vi "TCPGetVariableSets.vi"(1 "error in (no error)":errorcluster, 4 "connection ID":refnum<k5>) -> ()   [LabVIEW 2013]
uses:
  FBVarSet.ctl
  FBVar.ctl
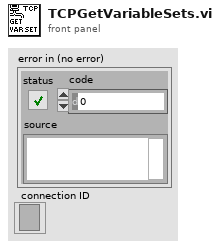
[diagram p1: front panel]
types:
  T1 = typedef "FBVarSet.ctl" = T2[]
  T2 = typedef "FBVar.ctl" = cluster{"Name":string, "Change DV":bool, "Default Value":dbl, "Change SF":bool, "Sequence Function":string, "Change II":bool, "Inform Igor":bool, "Change Seq.":bool, "Sequence":bool, "Change SV":bool, "String Value":string}
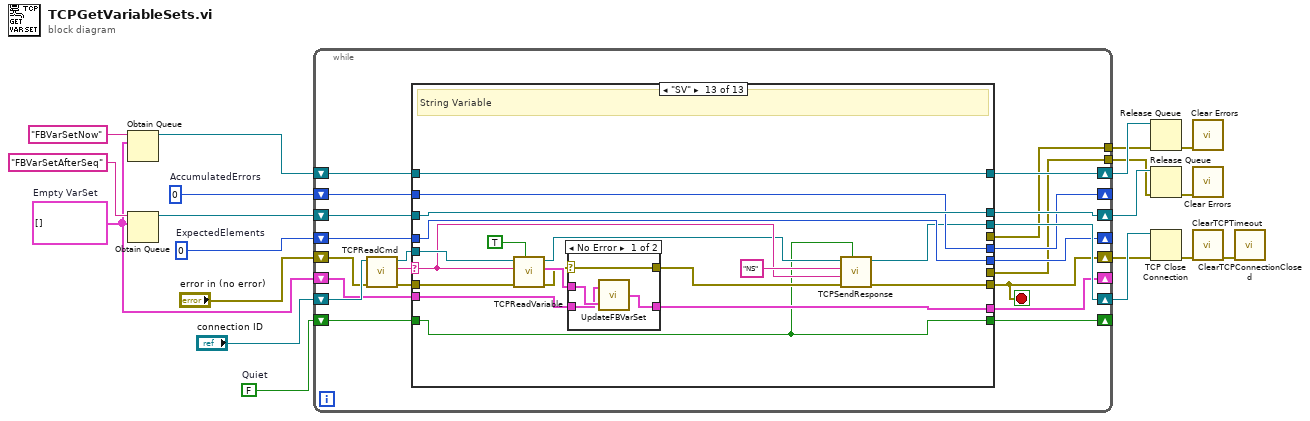
[diagram p0: block diagram]
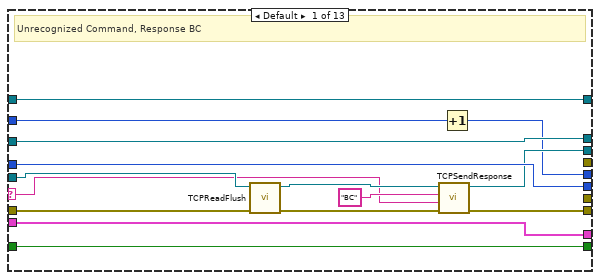
[diagram p2: hidden frame]
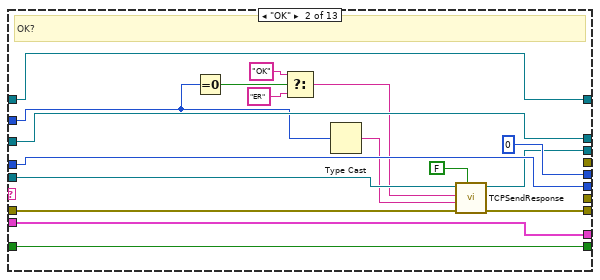
[diagram p3: hidden frame]
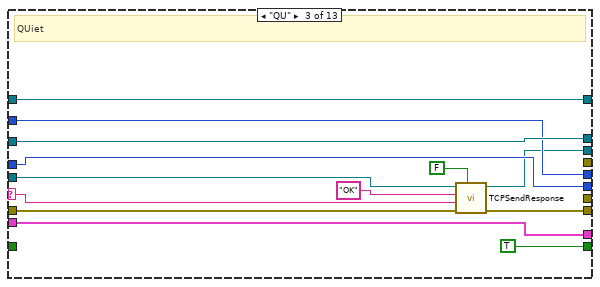
[diagram p4: hidden frame]
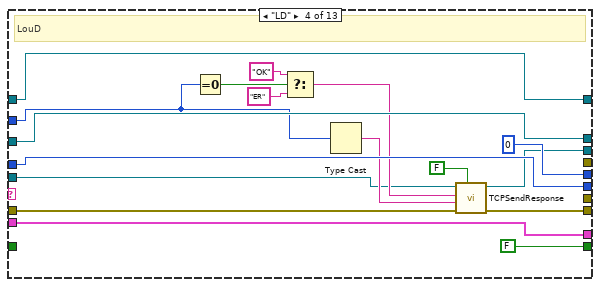
[diagram p5: hidden frame]
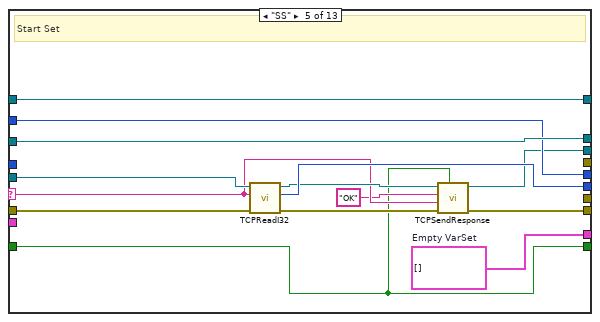
[diagram p6: hidden frame]
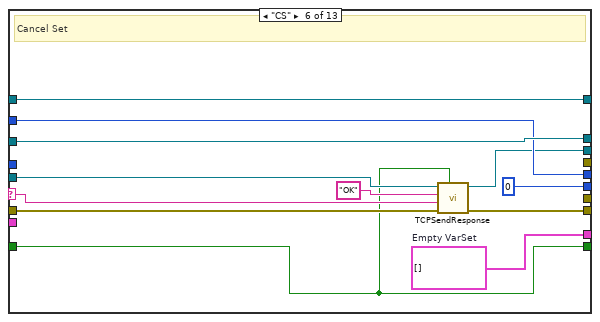
[diagram p7: hidden frame]
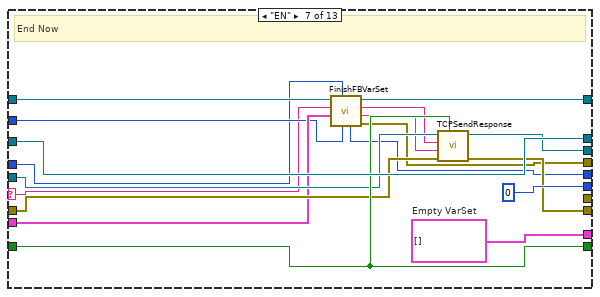
[diagram p8: hidden frame]
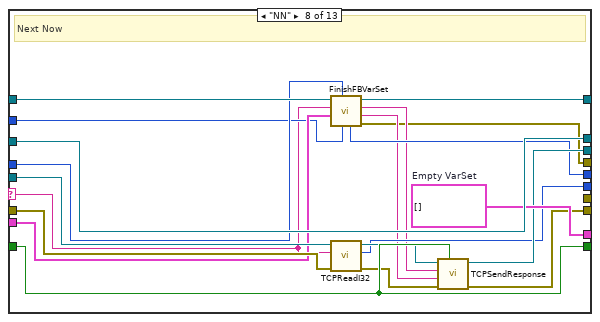
[diagram p9: hidden frame]
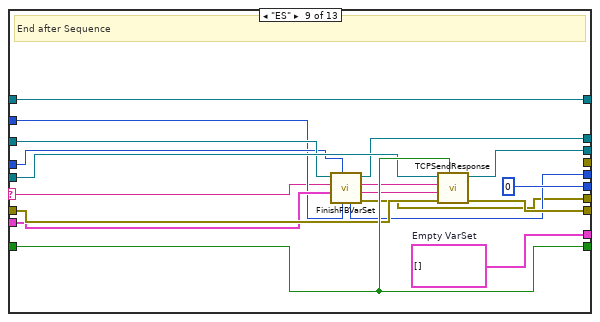
[diagram p10: hidden frame]
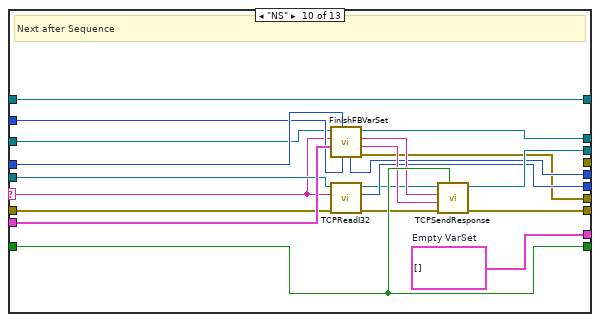
[diagram p11: hidden frame]
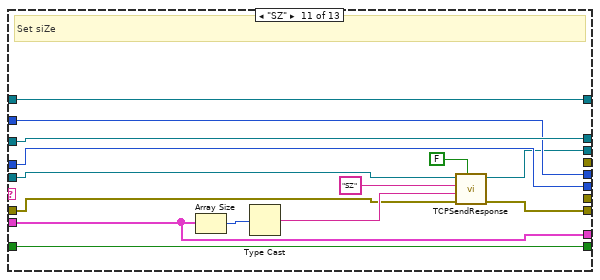
[diagram p12: hidden frame]
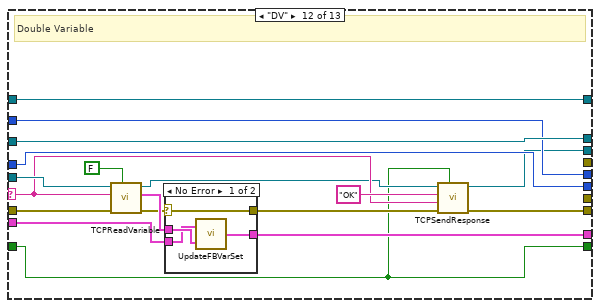
[diagram p13: hidden frame]
diagram:
  w3 = FALSE  # Quiet
  w4 = 0  # AccumulatedErrors
  w6 = T1 []  # Empty VarSet
  w5 = 0  # ExpectedElements
  n1 = Obtain Queue(name (unnamed)="FBVarSetNow", element data type=w6) -> (queue out=w17:refnum<queue>)  [unwired: 3 in, 2 out]
  n2 = Obtain Queue(name (unnamed)="FBVarSetAfterSeq", element data type=w6) -> (queue out=w11:refnum<queue>)  [unwired: 3 in, 2 out]
  n3 = while {
    shift-right: [w35] -> w20
    shift-left: "connection ID" -> [w41]
    shift-right: [w36] -> w16
    shift-left: w17 -> [w39]
    shift-right: [w23] -> w8
    shift-left: "error in (no error)" -> [w32]
    shift-right: [w28] -> _
    shift-left: w5 -> [w29]
    shift-right: [w38] -> w9
    shift-left: w11 -> [w40]
    shift-right: [w30] -> _
    shift-left: w6 -> [w31]
    shift-right: [w26] -> _
    shift-left: w4 -> [w27]
    shift-right: [w24] -> _
    shift-left: w3 -> [w25]
    tunnel: [w22] -> w2
    tunnel: [w21] -> w1
    stop <- w23 stop-if-true
    n4 = call "TCPReadCmd.vi"("error in (no error)"=w32, "connection ID"=w41) -> ("error out"=w33:errorcluster, "Command Code"=w37:string, "connection ID out"=w34:refnum<k5>)  [unwired: 7 in]
    n5 = case shown="\"SV\"" w37 {
      selector: w37 -> [w44 _ w74 _ w106 w125 w131 w149 w171 w188 _ w223 w247]
      tunnel: w40 -> [w56 w73 w86 w103 w117 w129 w147 w167 w176 w195 w219 w237 w261]
      tunnel: w39 -> [w55 w72 w85 w102 w116 w128 w138 w156 w178 w196 w218 w236 w260]
      tunnel: [w56 w73 w86 w103 w117 w129 w147 w167 w175 w194 w219 w237 w261] -> w38
      tunnel: [w55 w72 w85 w102 w116 w128 w137 w155 w178 w196 w218 w236 w260] -> w36
      tunnel: [w47 w61 w78 w88 w108 w121 w143 w164 w182 w200 w208 w221 w245] -> w35
      tunnel: w34 -> [w53 w62 w79 w92 w112 w123 w141 w159 w180 w190 w209 w228 w252]
      tunnel: w33 -> [w54 w63 w80 w91 w113 w126 w140 w158 w179 w193 w212 w227 w251]
      tunnel: [w48 w60 w77 w87 w107 w120 w144 w165 w183 w201 w211 w224 w249] -> w23
      tunnel: w31 -> [w52 w71 w84 w101 _ _ w139 w157 w177 w204 w206 w232 w256]
      tunnel: [w52 w71 w84 w101 w114 w119 w146 w166 w185 w205 w206 w231 w255] -> w30
      tunnel: w29 -> [w51 w70 w83 w100 _ _ w132 w154 w174 w203 w217 w235 w259]
      tunnel: [w51 w70 w83 w100 w111 0 ("I32 value") 0 ("I32 value") w160 0 ("I32 value") w191 w217 w235 w259] -> w28
      tunnel: w27 -> [w43 w67 w82 w90 w115 w127 w133 w153 w172 w202 w216 w234 w258]
      tunnel: [w42 0 ("AccumulatedErros") w82 0 ("AccumulatedErros") w115 w127 w134 w152 w173 w187 w216 w234 w258] -> w26
      tunnel: w25 -> [w50 w69 _ _ w104 w122 w142 w163 w181 w199 w215 w220 w244]
      tunnel: [w50 w69 TRUE ("Quiet") FALSE ("Quiet") w104 w122 w142 w163 w181 w199 w215 w220 w244] -> w24
      tunnel: [_ _ _ _ _ _ w130 w148 _ _ _ _ _] -> w22
      tunnel: [_ _ _ _ _ _ _ _ w168 w186 _ _ _] -> w21
      frame Default {
        # "Unrecognized Command, Response BC"
        n6 = call "TCPReadFlush.vi"("error in (no error)"=w54, "TCP Network Connection in"=w53) -> ("error out"=w49:errorcluster, "TCP Network Connection out"=w46:refnum<k5>)  [unwired: 8 in]
        n7 = call "TCPSendResponse.vi"("error in (no error)"=w49, "ResponseData"=w44, "ResponseCode"="BC" ("string"), "connection ID"=w46) -> ("error out"=w48:errorcluster, "connection ID out"=w47:refnum<k5>)  [unwired: 6 in]
        n8 = Increment(x=w43) -> (x+1=w42:i32)
      }
      frame "OK" {
        # "OK?"
        n9 = Equal To 0?(x=w67) -> (x = 0?=w66:bool)
        n10 = Select(t="OK" ("string"), s=w66, f="ER" ("string")) -> (s? t:f=w59:string)
        n11 = Type Cast(x=w67) -> (*(type *) &x=w58:string)  [unwired: 1 in]
        n12 = call "TCPSendResponse.vi"("Quiet"=FALSE, "error in (no error)"=w63, "ResponseData"=w58, "ResponseCode"=w59, "connection ID"=w62) -> ("error out"=w60:errorcluster, "connection ID out"=w61:refnum<k5>)  [unwired: 5 in]
      }
      frame "QU" {
        # "QUiet"
        n13 = call "TCPSendResponse.vi"("Quiet"=FALSE, "error in (no error)"=w80, "ResponseData"=w74, "ResponseCode"="OK", "connection ID"=w79) -> ("error out"=w77:errorcluster, "connection ID out"=w78:refnum<k5>)  [unwired: 5 in]
      }
      frame "LD" {
        # "LouD"
        n14 = Equal To 0?(x=w90) -> (x = 0?=w93:bool)
        n15 = Select(t="OK" ("string"), s=w93, f="ER" ("string")) -> (s? t:f=w96:string)
        n16 = Type Cast(x=w90) -> (*(type *) &x=w97:string)  [unwired: 1 in]
        n17 = call "TCPSendResponse.vi"("Quiet"=FALSE, "error in (no error)"=w91, "ResponseData"=w97, "ResponseCode"=w96, "connection ID"=w92) -> ("error out"=w87:errorcluster, "connection ID out"=w88:refnum<k5>)  [unwired: 5 in]
      }
      frame "SS" {
        w114 = T1 []  # Empty VarSet
        # "Start Set"
        n18 = call "TCPReadI32.vi"("error in (no error)"=w113, "command"=w106, "connection ID"=w112) -> ("error out"=w109:errorcluster, "I32 value"=w111:i32, "connection ID out"=w110:refnum<k5>)  [unwired: 6 in]
        n19 = call "TCPSendResponse.vi"("Quiet"=w104, "error in (no error)"=w109, "ResponseData"=w106, "ResponseCode"="OK" ("string"), "connection ID"=w110) -> ("error out"=w107:errorcluster, "connection ID out"=w108:refnum<k5>)  [unwired: 5 in]
      }
      frame "CS" {
        w119 = T1 []  # Empty VarSet
        # "Cancel Set"
        n20 = call "TCPSendResponse.vi"("Quiet"=w122, "error in (no error)"=w126, "ResponseData"=w125, "ResponseCode"="OK", "connection ID"=w123) -> ("error out"=w120:errorcluster, "connection ID out"=w121:refnum<k5>)  [unwired: 5 in]
      }
      frame "EN" {
        w146 = T1 []  # Empty VarSet
        # "End Now"
        n21 = call "FinishFBVarSet.vi"("AccumulatedErrors in"=w133, "ExpectedElements"=w132, "Finished VarSet"=w139, "Command"=w131, "Queue in"=w138) -> ("queue error out"=w130:errorcluster, "Response Data"=w135:string, "Response Code"=w136:string, "Queue out"=w137:refnum<queue>, "AccumulatedErrors out"=w134:i32)  [unwired: 2 in]
        n22 = call "TCPSendResponse.vi"("Quiet"=w142, "error in (no error)"=w140, "ResponseData"=w135, "ResponseCode"=w136, "connection ID"=w141) -> ("error out"=w144:errorcluster, "connection ID out"=w143:refnum<k5>)  [unwired: 5 in]
      }
      frame "NN" {
        w166 = T1 []  # Empty VarSet
        # "Next Now"
        n23 = call "FinishFBVarSet.vi"("AccumulatedErrors in"=w153, "ExpectedElements"=w154, "Finished VarSet"=w157, "Command"=w149, "Queue in"=w156) -> ("queue error out"=w148:errorcluster, "Response Data"=w150:string, "Response Code"=w151:string, "Queue out"=w155:refnum<queue>, "AccumulatedErrors out"=w152:i32)  [unwired: 2 in]
        n24 = call "TCPReadI32.vi"("error in (no error)"=w158, "command"=w149, "connection ID"=w159) -> ("error out"=w162:errorcluster, "I32 value"=w160:i32, "connection ID out"=w161:refnum<k5>)  [unwired: 6 in]
        n25 = call "TCPSendResponse.vi"("Quiet"=w163, "error in (no error)"=w162, "ResponseData"=w150, "ResponseCode"=w151, "connection ID"=w161) -> ("error out"=w165:errorcluster, "connection ID out"=w164:refnum<k5>)  [unwired: 5 in]
      }
      frame "ES" {
        w185 = T1 []  # Empty VarSet
        # "End after Sequence"
        n26 = call "FinishFBVarSet.vi"("AccumulatedErrors in"=w172, "ExpectedElements"=w174, "Finished VarSet"=w177, "Command"=w171, "Queue in"=w176) -> ("queue error out"=w168:errorcluster, "Response Data"=w170:string, "Response Code"=w169:string, "Queue out"=w175:refnum<queue>, "AccumulatedErrors out"=w173:i32)  [unwired: 2 in]
        n27 = call "TCPSendResponse.vi"("Quiet"=w181, "error in (no error)"=w179, "ResponseData"=w170, "ResponseCode"=w169, "connection ID"=w180) -> ("error out"=w183:errorcluster, "connection ID out"=w182:refnum<k5>)  [unwired: 5 in]
      }
      frame "NS" {
        w205 = T1 []  # Empty VarSet
        # "Next after Sequence"
        n28 = call "FinishFBVarSet.vi"("AccumulatedErrors in"=w202, "ExpectedElements"=w203, "Finished VarSet"=w204, "Command"=w188, "Queue in"=w195) -> ("queue error out"=w186:errorcluster, "Response Data"=w197:string, "Response Code"=w198:string, "Queue out"=w194:refnum<queue>, "AccumulatedErrors out"=w187:i32)  [unwired: 2 in]
        n29 = call "TCPReadI32.vi"("error in (no error)"=w193, "command"=w188, "connection ID"=w190) -> ("error out"=w192:errorcluster, "I32 value"=w191:i32, "connection ID out"=w189:refnum<k5>)  [unwired: 6 in]
        n30 = call "TCPSendResponse.vi"("Quiet"=w199, "error in (no error)"=w192, "ResponseData"=w197, "ResponseCode"=w198, "connection ID"=w189) -> ("error out"=w201:errorcluster, "connection ID out"=w200:refnum<k5>)  [unwired: 5 in]
      }
      frame "SZ" {
        # "Set siZe"
        n31 = Array Size(array=w206) -> (size(s)=w207:i32)
        n32 = Type Cast(x=w207) -> (*(type *) &x=w213:string)  [unwired: 1 in]
        n33 = call "TCPSendResponse.vi"("Quiet"=FALSE, "error in (no error)"=w212, "ResponseData"=w213, "ResponseCode"="SZ", "connection ID"=w209) -> ("error out"=w211:errorcluster, "connection ID out"=w208:refnum<k5>)  [unwired: 5 in]
      }
      frame "DV" {
        # "Double Variable"
        n34 = call "TCPReadVariable.vi"("String Var?"=FALSE, "error in (no error)"=w227, "command"=w223, "connection ID"=w228) -> ("error out"=w230:errorcluster, "Variable"=w233:T2, "connection ID out"=w222:refnum<k5>)  [unwired: 5 in]
        n35 = case shown="No Error" w230 {
          selector: w230 -> [w238 w243]
          tunnel: w233 -> [w241 _]
          tunnel: w232 -> [w240 w242]
          tunnel: [w239 w242] -> w231
          tunnel: [w238 w243] -> w225
          frame No Error {
            n36 = call "UpdateFBVarSet.vi"("Variable"=w241, "CurrentVarSet"=w240) -> ("UpdatedVarSet"=w239:T1)
          }
          frame Error {
          }
        }
        n37 = call "TCPSendResponse.vi"("Quiet"=w220, "error in (no error)"=w225, "ResponseData"=w223, "ResponseCode"="OK" ("string"), "connection ID"=w222) -> ("error out"=w224:errorcluster, "connection ID out"=w221:refnum<k5>)  [unwired: 5 in]
      }
      frame "SV" {
        # "String Variable"
        n38 = call "TCPReadVariable.vi"("String Var?"=TRUE, "error in (no error)"=w251, "command"=w247, "connection ID"=w252) -> ("error out"=w254:errorcluster, "Variable"=w257:T2, "connection ID out"=w246:refnum<k5>)  [unwired: 5 in]
        n39 = case shown="No Error" w254 {
          selector: w254 -> [w262 w267]
          tunnel: w257 -> [w265 _]
          tunnel: w256 -> [w264 w266]
          tunnel: [w263 w266] -> w255
          tunnel: [w262 w267] -> w248
          frame No Error {
            n40 = call "UpdateFBVarSet.vi"("Variable"=w265, "CurrentVarSet"=w264) -> ("UpdatedVarSet"=w263:T1)
          }
          frame Error {
          }
        }
        n41 = call "TCPSendResponse.vi"("Quiet"=w244, "error in (no error)"=w248, "ResponseData"=w247, "ResponseCode"="NS" ("string"), "connection ID"=w246) -> ("error out"=w249:errorcluster, "connection ID out"=w245:refnum<k5>)  [unwired: 5 in]
      }
    }
  }
  n42 = Release Queue(queue=w16, error in (no error)=w2) -> (error out=w15:errorcluster)  [unwired: 1 in, 2 out]
  n43 = Release Queue(queue=w9, error in (no error)=w1) -> (error out=w10:errorcluster)  [unwired: 1 in, 2 out]
  n44 = TCP Close Connection(connection ID=w20, error in (no error)=w8) -> (error out=w14:errorcluster)  [unwired: 1 in, 1 out]
  n45 = call <vilib>:"Clear Errors.vi"("error in (no error)"=w15) -> ()  [unwired: 6 in, 1 out]
  n46 = call <vilib>:"Clear Errors.vi"("error in (no error)"=w10) -> ()  [unwired: 6 in, 1 out]
  n47 = call "ClearTCPTimeout.vi"("error in (no error)"=w14) -> ("error out"=w13:errorcluster)  [unwired: 9 in, 1 out]
  n48 = call "ClearTCPConnectionClosed.vi"("error in (no error)"=w13) -> ()  [unwired: 9 in, 2 out]
